vi "ATF Storage-Append WF_AIV.vi"(7 "Samples":i32=10, 9 "Data input":waveform(dbl)[](array[waveform]), 10 "Data_init":dbl[][](array[numeric]), 11 "Waveform_Init":timestamp[][](array[timestamp])) -> (1 "Data out":waveform(dbl)[](array[waveform]), 2 "Data_SR":dbl[][](array[numeric]), 3 "WF_SR":timestamp[][](array[timestamp]))   [LabVIEW 2022 SP3]
panel:
  in  "size":i32
  out "x-y 2":u32
  out "x-y":u32
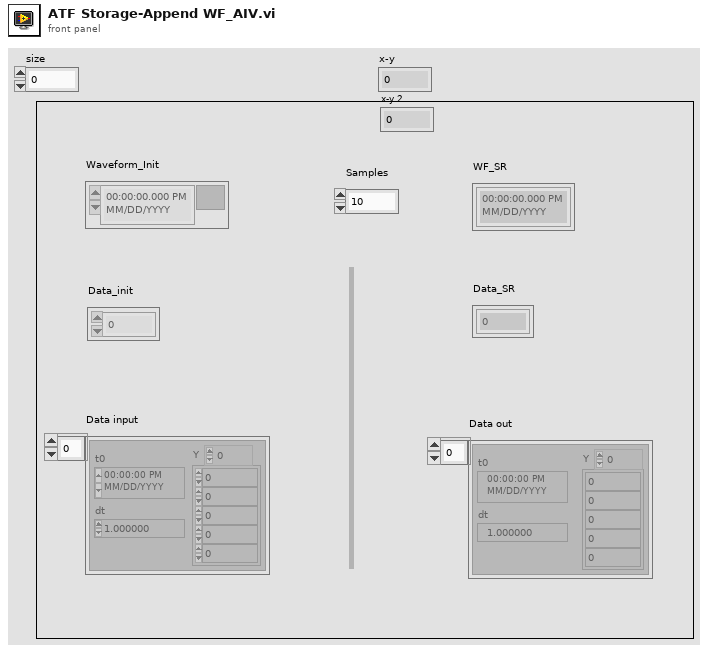
[diagram p1: front panel]
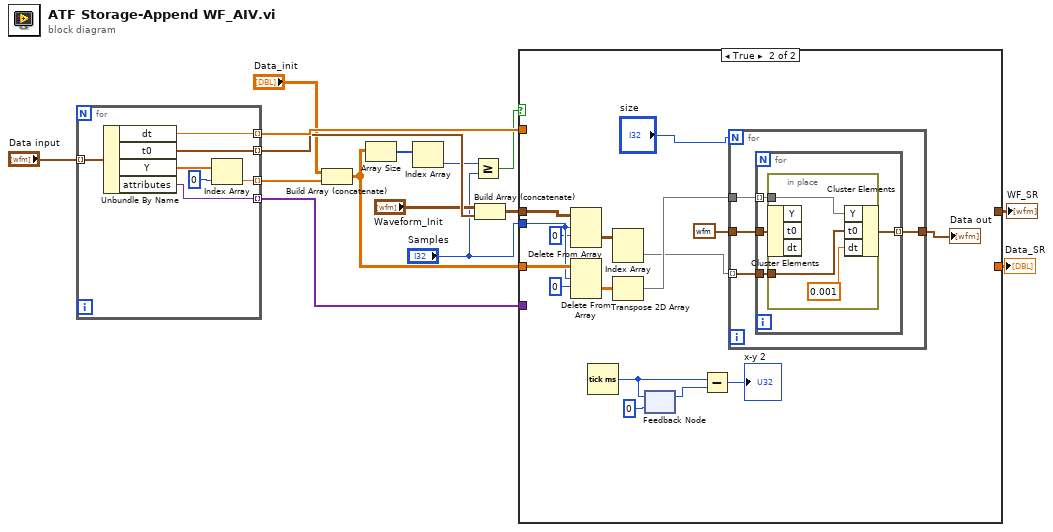
[diagram p0: block diagram]
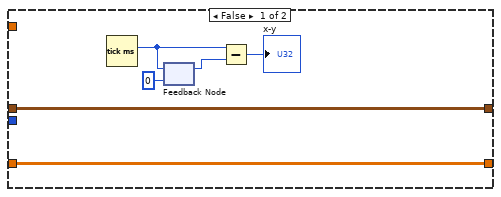
[diagram p2: hidden frame]
diagram:
  n1 = for {
    tunnel: "Data input" -> [w22] mode=indexing
    tunnel: [w20] -> w3 mode=indexing
    tunnel: [w18] -> w11 mode=indexing
    tunnel: [w17] -> w14 mode=indexing
    tunnel: [w16] -> w15 mode=indexing
    n2 = Unbundle By Name(w22) -> ("dt"=w16:dbl, "t0"=w18:timestamp, "Y"=w21:dbl[], "attributes"=w17:variant)
    n3 = Index Array(array=w21, index=0) -> (element=w20:dbl)
  }
  n4 = Build Array (concatenate)("Data_init", w3) -> (w6:dbl[][])
  n5 = Array Size(array=w6) -> (size(s)=w4:i32[])
  n6 = Index Array(array=w4) -> (element=w5:i32)  [unwired: 1 in]
  n7 = Greater Or Equal?(x=w5, y="Samples") -> (x >= y?=w8:bool)
  n8 = Build Array (concatenate)("Waveform_Init", w11) -> (w12:timestamp[][])
  n9 = case shown="True" w8 {
    tunnel: w6 -> [w28 w44]
    tunnel: [w28 _] -> w7
    tunnel: w12 -> [w27 w42]
    tunnel: [w27 _] -> w13
    tunnel: w14 -> [_ _]
    tunnel: w15 -> [_ _]
    tunnel: "Samples" -> [_ w40]
    frame False {
      n10 = Tick Count (ms)() -> (millisecond timer value=w26:u32)
      n11 = feedback-in #1(w26) -> ()
      n12 = feedback #1(u32 0 ("millisecond timer value")) -> (w25:u32)
      n13 = Subtract(x=w26, y=w25) -> (x-y=→"x-y":u32)
    }
    frame True {
      n14 = Delete From Array(array=w42, length=w40, index (row)=0) -> (deleted portion=w41:timestamp[][])  [unwired: 1 in, 1 out]
      n15 = Delete From Array(array=w44, length=w40, index (row)=0) -> (deleted portion=w43:dbl[][])  [unwired: 1 in, 1 out]
      n16 = Tick Count (ms)() -> (millisecond timer value=w37:u32)
      n17 = Index Array(array=w41) -> (element=w30:timestamp[])  [unwired: 2 in]
      n18 = Transpose 2D Array(2D array=w43) -> (transposed array=w31:dbl[][])
      n19 = feedback #2(u32 0 ("millisecond timer value")) -> (w36:u32)
      n20 = feedback-in #2(w37) -> ()
      n21 = Subtract(x=w37, y=w36) -> (x-y=→"x-y 2":u32)
      n22 = for {
        N: "size" -> [_]
        tunnel: waveform(dbl) {"t0"=timestamp(0 s since 1904-01-01), "dt"=0.001, "Y"=[]} ("Waveform") -> [w48]
        tunnel: [w47] -> w29
        tunnel: w31 -> [w46]
        tunnel: w30 -> [w45] mode=indexing
        n23 = for {
          tunnel: [w51] -> w47 mode=indexing
          tunnel: w48 -> [w52]
          tunnel: w46 -> [w50] mode=indexing
          tunnel: w45 -> [w49]
          n24 = in-place {
            in-place-border: w50 -> [w55]
            in-place-border: w49 -> [w54]
            n25 = in-place-cluster #3(w52) -> ()  [unwired: 3 out]
            n26 = in-place-cluster #3("Y"=w55, "t0"=w54, "dt"=0.001) -> (w51:waveform(dbl))
          }
        }
      }
      "Data out" <- w29
    }
  }
  "WF_SR" <- w13
  "Data_SR" <- w7
